vi "Read File Folder.vi"(8 "error in (no error)":errorcluster, 11 "SystemLink File configuration in":refnum<class "SystemLink File configuration.lvclass">) -> (0 "error out":errorcluster, 2 "File Folder":string, 3 "SystemLink File configuration out":refnum<class "SystemLink File configuration.lvclass">)   [LabVIEW 2015, in "SystemLink File configuration.lvclass"]
uses:
  SystemLink File configuration.lvclass
  SystemLink File configuration.lvclass/SystemLink File configuration.ctl
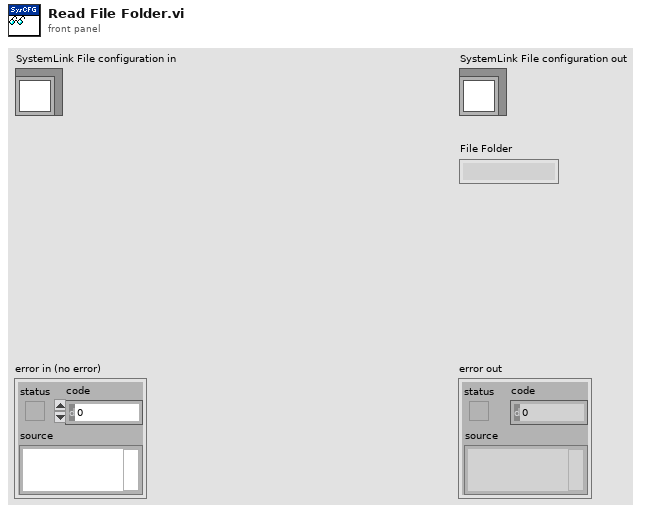
[diagram p1: front panel]
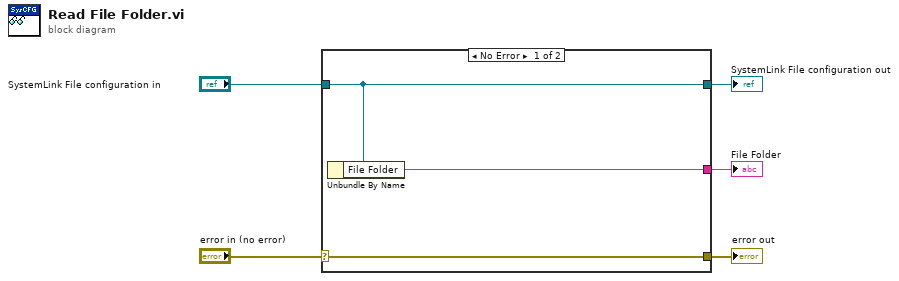
[diagram p0: block diagram]
diagram:
  n1 = case shown="No Error" "error in (no error)" {
    selector: "error in (no error)" -> [w8 w9]
    tunnel: [w8 w9] -> w4
    tunnel: [w7 w10] -> w2
    tunnel: "SystemLink File configuration in" -> [w7 w10]
    tunnel: [w6 _] -> w1
    frame No Error {
      n2 = Unbundle By Name(w7) -> ("File Folder"=w6:string)
    }
    frame Error {
    }
  }
  "error out" <- w4
  "SystemLink File configuration out" <- w2
  "File Folder" <- w1
